vi "valve_control_output.vi"(0 "STOP! Refnum":refnum<vi>, 2 "Voltage Arr Refnum":refnum<vi>, 3 "PG channel":tag="cDAQ1Mod3/ao1", 4 "Liquid channel":tag="cDAQ1Mod4/ao3", 5 "Vapor channel":tag="cDAQ1Mod4/ao2") -> ()   [LabVIEW 2017]
uses:
  <vilib>/DAQmx/write.llb/DAQmx Write (Analog 1D DBL NChan 1Samp).vi
  <vilib>/DAQmx/create/channels.llb/DAQmx Create Channel (AO-Voltage-Basic).vi
  <vilib>/DAQmx/miscellaneous.llb/DAQmx Fill In Error Info.vi
  <resource>/objmgr/daqmx.rc
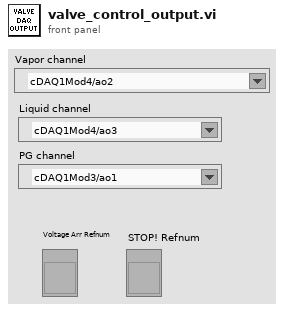
[diagram p1: front panel]
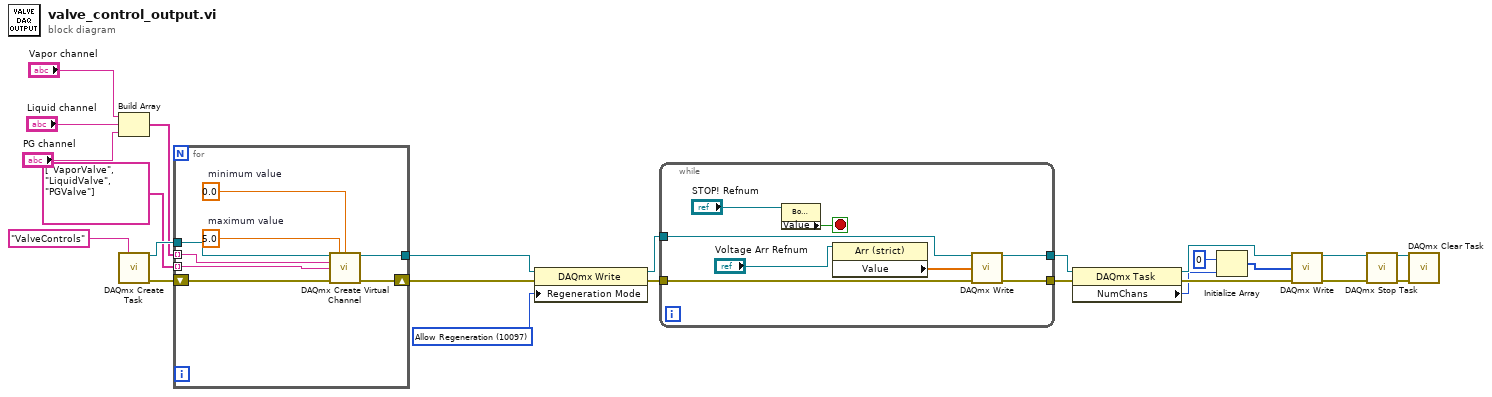
[diagram p0: block diagram]
diagram:
  w18 = 10097 items=["Allow Regeneration"=10097, "Do Not Allow Regeneration"=10158] ("RegenMode")
  n1 = Build Array("Vapor channel", "Liquid channel", "PG channel") -> (w19:tag[])
  n2 = call <vilib>:"DAQmx Create Task.vi"("new task name"="ValveControls") -> ("task out"=w24:refnum<k21>, "error out"=w23:errorcluster)  [unwired: 13 in]
  n3 = for {
    tunnel: w24 -> [w32]
    shift-right: [w25] -> w14
    shift-left: w23 -> [w31]
    tunnel: string[] ["VaporValve", "LiquidValve", "PGValve"] -> [w30] mode=indexing
    tunnel: w19 -> [w29] mode=indexing
    tunnel: [w26] -> w15
    w27 = 0.0  # minimum value
    w28 = 5.0  # maximum value
    n4 = call-poly <vilib>:"DAQmx Create Virtual Channel.vi"("task in"=w32, "maximum value"=w28, "minimum value"=w27, "physical channels"=w29, "name to assign"=w30, "error in"=w31) -> ("task out"=w26:refnum<k21>, "error out"=w25:errorcluster)  [unwired: 8 in]
  }
  n5 = property class="DAQmx Write"(reference=w15, error in=w14, "Regeneration Mode"=w18) -> (reference out=w12:refnum<k21>, error out=w13:errorcluster)
  n6 = while {
    tunnel: w12 -> [w35]
    tunnel: [w34] -> w5
    tunnel: w13 -> [w38]
    tunnel: [w33] -> w8
    stop <- w39 stop-if-true
    n7 = property class="Bool (strict)"(reference="STOP! Refnum") -> ("Value"=w39:bool)  [unwired: 1 in, 2 out]
    n8 = property class="Arr (strict)"(reference="Voltage Arr Refnum") -> ("Value"=w36:dbl[])  [unwired: 1 in, 2 out]
    n9 = call-poly <vilib>:"DAQmx Write.vi"("task/channels in"=w35, "data"=w36, "error in"=w38) -> ("task out"=w34:refnum<k21>, "error out"=w33:errorcluster)  [unwired: 10 in, 1 out]
  }
  n10 = property class="DAQmx Task"(reference=w5, error in=w8) -> (reference out=w4:refnum<k21>, error out=w3:errorcluster, "NumChans"=w2:u32)
  n11 = Initialize Array(u32 0 ("element"), w2) -> (w6:u32[])
  n12 = call-poly <vilib>:"DAQmx Write.vi"("task/channels in"=w4, "data"=w6, "error in"=w3) -> ("task out"=w10:refnum<k21>, "error out"=w9:errorcluster)  [unwired: 10 in, 1 out]
  n13 = call <vilib>:"DAQmx Stop Task.vi"("task/channels in"=w10, "error in"=w9) -> ("task out"=w17:refnum<k21>, "error out"=w16:errorcluster)  [unwired: 12 in]
  n14 = call <vilib>:"DAQmx Clear Task.vi"("task in"=w17, "error in"=w16) -> ()  [unwired: 13 in, 1 out]
